vi "FXP_AFMss_MPC_singleAxis_N22.vi"() -> ()   [LabVIEW 2017]
uses:
  fpga_fp_interface_lib/fpga_interface_types/boolean_indicators.ctl
  fgm_pipiline/quadProgParams_pipe.ctl
  typeDefs/FXPControlParams_distEst.ctl
  <vilib>/rvi/eio/common/nirviEmuClasses.ctl
  <vilib>/Platform/TimedLoop/XDataNode/timing_clust.ctl
  <vilib>/Platform/TimedLoop/XDataNode/nitl_modes.ctl
  <vilib>/Platform/TimedLoop/XDataNode/wakeup.ctl
  <vilib>/rvi/Emulation/niFpgaSctlEmulationGetInTimedLoop.vi
  <vilib>/rvi/Emulation/niFpgaProcessEmulError.vi
  <vilib>/rvi/eio/common/nirviEmuTemplateMethod_errors.vi
  <vilib>/rvi/Emulation/niFpgaGetClockAttributes.vi
  <vilib>/rvi/Emulation/niFpgaEmulationReportErrorSimple.vi
  <vilib>/rvi/Emulation/niFpgaCriticalErrorInLSC.vi
  <vilib>/rvi/Memory/Memory_Emulation/nirvimemoryFastEmulation.vi
  <vilib>/rvi/Memory/Memory_Emulation/nirvimemoryEmulation.vi
  <vilib>/rvi/Emulation/niFpgaEmulationIsFPGAContextNoSignature.vi
  <vilib>/rvi/DataTransferAndStorage/Container/Common/niFpgaContainerGetUniqueNameForEmu.vi
  <vilib>/rvi/errors/nirviReportUnexpectedCaseInternalError (U32).vi
  <vilib>/rvi/interface/RandomDataEmulation/niFpgaRandomDataHandleErrors.vi
  <vilib>/eio/EIOGrowableMethodNode/genericMethod/EIOGrowableMethodNode.xnode
  <vilib>/rvi/eio/nirviEIOMethodImplementation/nirviEIOMethodImplementation.xnode
  <vilib>/rvi/eio/nirviErrorMerge/nirviErrorMerge.xnode
  <vilib>/eio/EIONode/EIONode.xnode
  <vilib>/Platform/TimedLoop/XDataNode/XDataNode.xnode
  <vilib>/rvi/DataTransferAndStorage/Container/XNode/niFpgaContainer.xnode
  <vilib>/rvi/interface/RandomDataEmulation/nirviRandomDataFpgaReadWriteTemplate.vi
  <vilib>/rvi/FXPMathLib/FxpSub/XNode/nifxpmath_Sub.xnode
  <vilib>/Platform/TimedLoop/XDataNode/XDNodeRunTimeDep.lvlib
  <vilib>/rvi/FXPMathLib/sim/FxpSim.dll
panel:
  in  "N_sat":i32
  in  "sat_d_s":fxp<+/-,16,5>[](array[numeric])=[0.0, 0.0, 0.0, 0.0, 0.0, 0.0, 0.0]
  in  "sat_w_s":fxp<+/-,16,5>[](array[numeric])=[0.0, 0.0, 0.0, 0.0, 0.0, 0.0, 0.0]
  out "fpga_debug":bool
  out "fpga_debug":bool
  in  "N_hyst":i32
  in  "w_s":fxp<+/-,16,5>[](array[numeric])=[0.0, 0.0, 0.0, 0.0, 0.0, 0.0, 0.0]
  in  "r_s":fxp<+/-,16,5>[](array[numeric])=[0.0, 0.0, 0.0, 0.0, 0.0, 0.0, 0.0]
  out "Ipow fast":fxp<+/-,16,5>
  in  "Num":sgl[](array[numeric])=[-0.00254, 0.000408, 0.00295, 0.0, 0.0, 0.0, 0.0, 0.0, 0.0]
  in  "Den":sgl[](array[numeric])=[0.982758, -1.98194, 1.0, 0.0, 0.0, 0.0, 0.0, 0.0, 0.0]
  in  "TF Order":i32=2
  out "y_ref":sgl
  in  "ControlParams_distEst":T1={"umax"=3.0, "Ns_obs/cntrl"=0, "ref_f_VEC"=[0.0, 0.0], "du_max"=0.0}
  in  "QP_params":T2={"maxIter"=0, "nuN"=24, "Ns_mpc"=0, "-beta"=-0.9987945556640625, "beta+1"=1.9987945556640625}
  out "Matrix FIFO \nTimeOut":bool
  out "u_k":fxp<+/-,32,5>
  out "boolean  indicators":T3
  out "x-x(0)":fxp<+/-,18,5>
  out "y-axis fast":fxp<+/-,16,5>
  out "x(0)":fxp<+/-,16,5>
  out "LoopTicks2":u32
  out "Error Out":errorcluster
  out "x-axis fast":fxp<+/-,16,5>
  out "AI Timed Out":bool
  out "Stopped":bool
  in  "Settle Ticks":i16=1000
  in  "iters":i32=1
  in  "ymax":fxp<+/-,32,16>=4.0
  in  "TsTicks":i16
  out "Loop Ticks (benchmark)":i16
  out "NS_O/C":u8=2
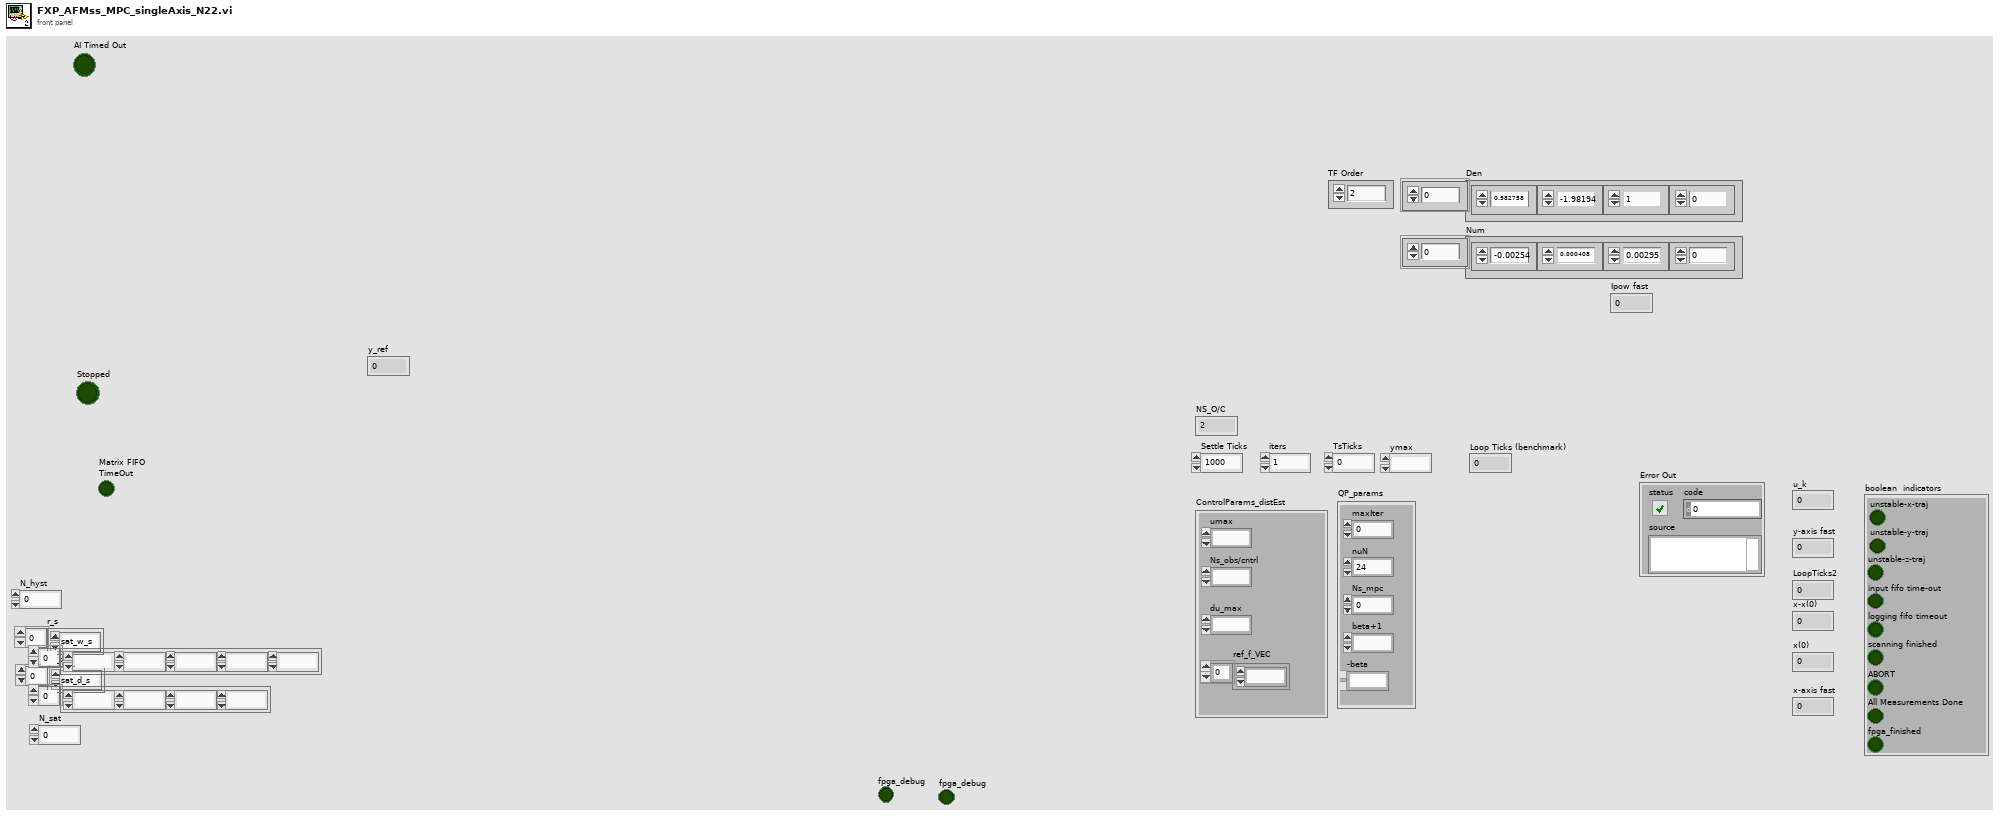
[diagram p1: front panel]
types:
  T1 = typedef "FXPControlParams_distEst.ctl" = cluster{"umax":fxp<+/-,18,5>, "Ns_obs/cntrl":u8, "ref_f_VEC":fxp<+/-,32,5>[], "du_max":fxp<+/-,18,5>}
  T2 = typedef "quadProgParams_pipe.ctl" = cluster{"maxIter":u16, "nuN":u16, "Ns_mpc":u16, "-beta":fxp<+/-,18,2>, "beta+1":fxp<+/-,18,2>}
  T3 = typedef "boolean_indicators.ctl" = cluster{"unstable-z-traj":bool, "input fifo time-out":bool, "logging fifo timeout":bool, "scanning finished":bool, "unstable-x-traj":bool, "unstable-y-traj":bool, "ABORT":bool, "All Measurements Done":bool, "fpga_finished":bool}
  T4 = typedef "nirviEmuClasses.ctl" = enum16{"IO Read", "IO Write", "Method", "Property Read", "Property Write"}
  T5 = typedef "XDNodeRunTimeDep.lvlib/timing_clust.ctl" = cluster{"Expected End [f-1]":u64, "Actual End [f-1]":u64, "Finished Late? [f-1]":bool, "Expected End [i-1]":u64, "Actual End [i-1]":u64, "Finished Late? [i-1]":bool, "Expected Start [i]":u64, "Actual Start [i]":u64, "Expected Start [f]":u64, "Actual Start [f]":u64, "Source Name":string, "Structure Name":string, "Period":i64, "Deadline":i64, "Offset":i64, "Start":i64, "Priority":i32, "Timeout":i32, "Mode":T6, "Wakeup Reason":T7, "Error":errorcluster, "Source Type":string, "Secondary Source Type":string, "Global End Time":u64, "Global Start Time":u64, "Frame Duration":u64, "Iteration Duration":u64, "Assigned CPU":i32, "I/O Scan Engine Mode":u32}
  T6 = typedef "XDNodeRunTimeDep.lvlib/nitl_modes.ctl" = enum32{"No Change", "Process missed periods, maintain original phase", "Discard missed periods, maintain original phase", "Process missed periods, ignore original phase", "Discard missed periods, ignore original phase"}
  T7 = typedef "XDNodeRunTimeDep.lvlib/wakeup.ctl" = enum32{"Normal", "Aborted", "Asynchronous wakeup", "Timing source error", "Timed loop error", "Timeout"}
  T8 = typedef "x_vec_type.ctl" = fxp<+/-,32,6>[]
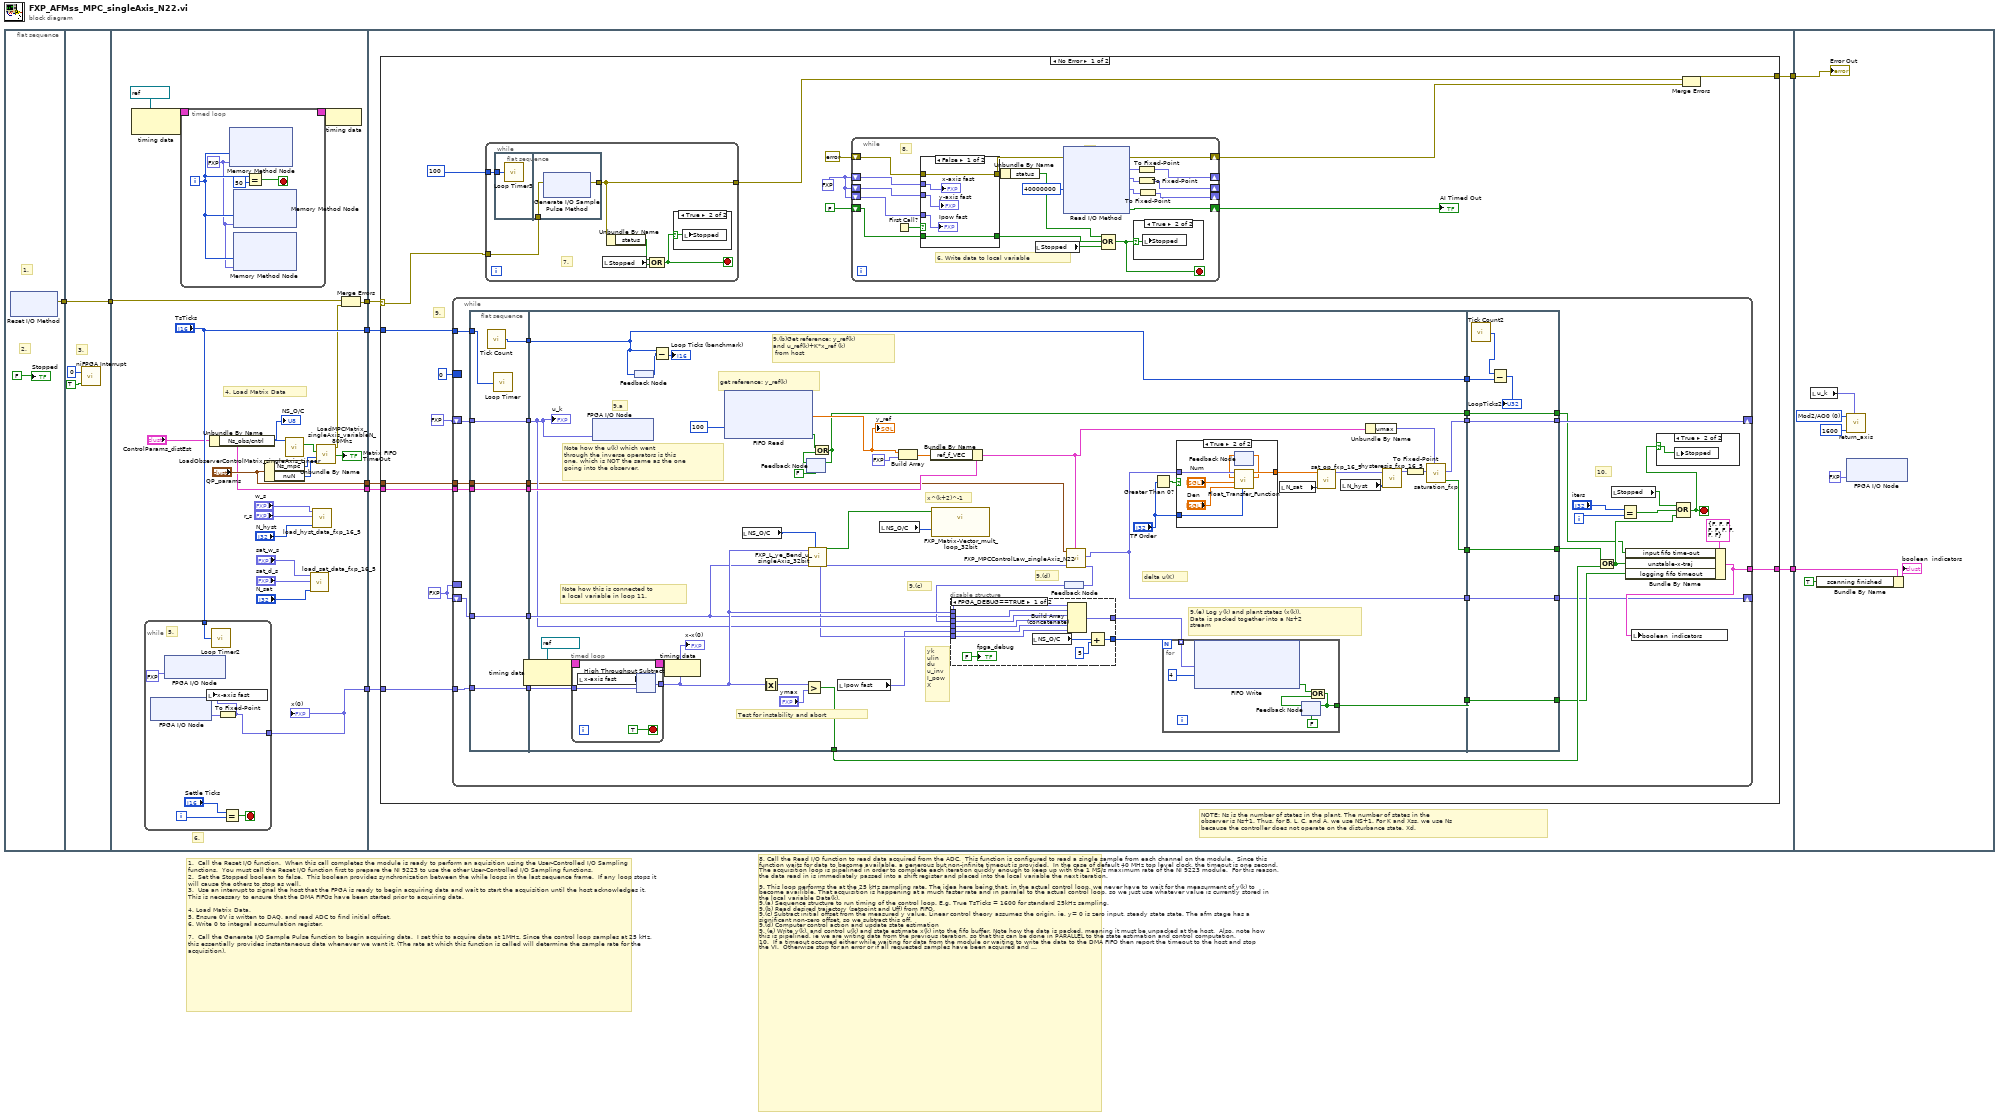
[diagram p0: block diagram]
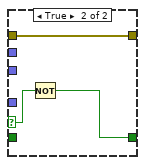
[diagram p2: hidden frame]
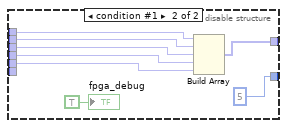
[diagram p6: hidden frame]
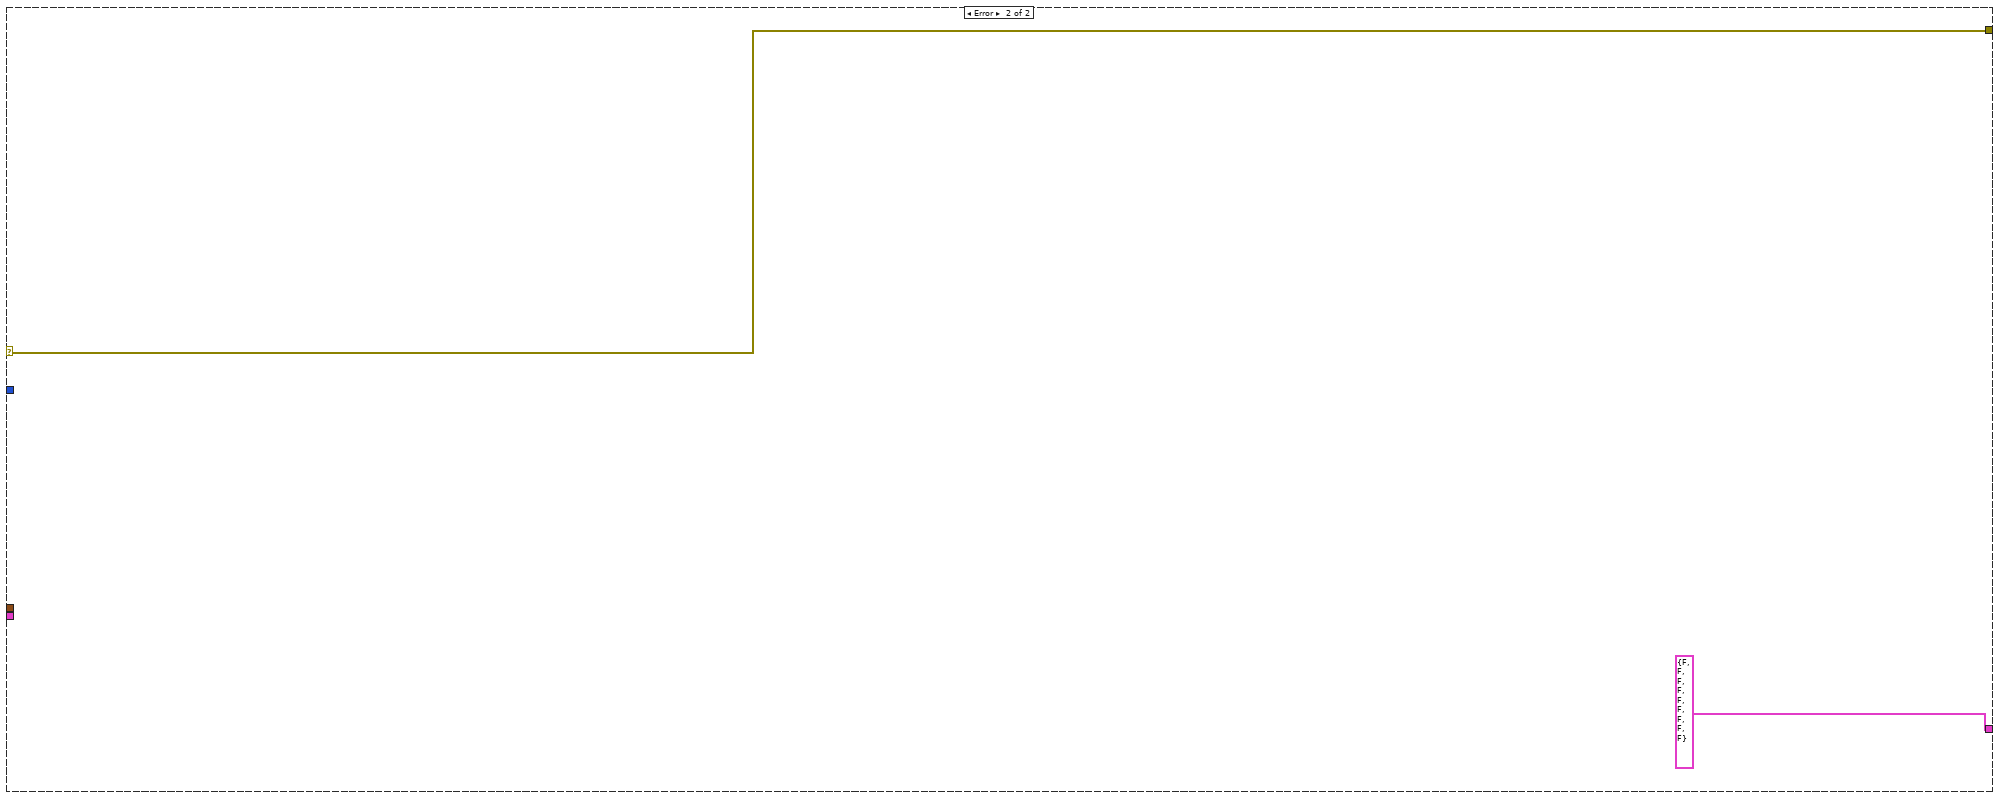
[diagram p8: hidden frame]
diagram:
  # "8. Call the Read I/O function to read data acquired from the ADC.  This function is configured to read a single sample from each channel on the module.  Since this function waits for data to become available, a generous but non-infinite timeout is provided.  In the case of default 40 MHz top level clock, the timeout is one second.  The acquisition loop is pipelined in order to complete each iteration quickly enough to keep up with the 1 MS/s maximum rate of the NI 9223 module.  For this reason, the data read in is immediately passed into a shift register and placed into the local variable the next iteration.\n\n9. This loop performs the at the 25 kHz sampling rate. The idea here being that, in the actual control loop, we never have to wait for the measurment of y(k) to become availible. That acquisition is happening at a much faster rate and in parralel to the actual control loop, so we just use whatever value is currently stored in the local variable Data(k).\n9.(a) Sequence structure to run timing of the control loop. E.g. True TsTicks = 1600 for standard 25kHz sampling.\n9.(b) Read desired trajectory (setpoint and Uff) from FIFO.\n9.(c) Subtract initial offset from the measured y value. Linear control theory assumes the origin, ie, y= 0 is zero input, steady state state. The afm stage has a significant non-zero offset, so we subtract this off.\n9.(d) Computer control action and update state estimation\n9. (e) Write y(k), and control u(k) and state estimate x(k) into the fifo buffer. Note how the data is packed, meaning it must be unpacked at the host.  Also, note how this is pipelined, ie we are writing data from the previous iteration, so that this can be done in PARALLEL to the state estimation and control computation.  \n10.  If a timeout occurred either while waiting for data from the module or waiting to write the data to the DMA FIFO then report the timeout to the host and stop the VI.  Otherwise stop for an error or if all requested samples have been acquired and placed into the DMA FIFO or if the controll law has detected instability.\n\n11. WRITE  TO DAQ. Note how the output of the control law is connected to loop 11 through a local variable."
  # "1.  Call the Reset I/O function.  When this call completes the module is ready to perform an aquisition using the User-Controlled I/O Sampling functions.  You must call the Reset I/O function first to prepare the NI 9223 to use the other User-Controlled I/O Sampling functions.\n2.  Set the Stopped boolean to false.  This boolean provides synchronization between the while loops in the last sequence frame.  If any loop stops it will cause the others to stop as well.\n3.  Use an interrupt to signal the host that the FPGA is ready to begin acquiring data and wait to start the acquisition until the host acknowledges it.  This is necessary to ensure that the DMA FIFOs have been started prior to acquiring data.\n\n4. Load Matrix Data.\n5. Ensure 0V is written to DAQ, and read ADC to find initial offset.\n6. Write 0 to integral accumulation register.\n\n7.  Call the Generate I/O Sample Pulse function to begin acquiring data.  I set this to acquire data at 1MHz. Since the control loop samples at 25 kHz, this essentially provides instantaneous data whenever we want it. (The rate at which this function is called will determine the sample rate for the acquisition)."
  n1 = flat-sequence {
    tunnel: [w10] -> w4
    tunnel: [w56] -> w5
    tunnel: w4 -> [w56]
    tunnel: ["TsTicks"] -> w9
    tunnel: [w79] -> w8
    tunnel: ["ControlParams_distEst"] -> w7
    tunnel: [w73] -> w6
    tunnel: w5 -> [w72]
    tunnel: ["QP_params"] -> w1
    tunnel: w9 -> [w103]
    tunnel: w8 -> [w102]
    tunnel: w7 -> [w101]
    tunnel: w6 -> [w100]
    tunnel: [w99] -> w3
    tunnel: [w98] -> w2
    tunnel: w1 -> [w97]
    tunnel: w3 -> [w495]
    tunnel: w2 -> [w493]
    frame #0 {
      # "2."
      # "1."
      n2 = xnode "Reset I/O Method"() -> ("error out"=w10:errorcluster)  [unwired: 2 in, 1 out]
      "Stopped" <- FALSE ("Stopped")
    }
    frame #1 {
      # "3."
      n3 = call <vilib>:"niFPGA Interrupt.vi"("Wait Until Cleared (F)"=TRUE, "IRQ Number (0)"=u8 0) -> ()  [unwired: 1 in]
    }
    frame #2 {
      # "6."
      # "4. Load Matrix Data"
      n4 = node-c288(refnum<k21> "80MHz" ("Source Name")) -> (w77:T5)
      n5 = while {
        tunnel: [w94] -> w79
        tunnel: "TsTicks" -> [w96]
        i -> [w90]
        stop <- w92 stop-if-true
        # "5."
        n6 = xnode "FPGA I/O Node"() -> ("Mod2/AI0"=w95:fxp<+/-,24,5>)  [unwired: 1 in, 1 out]
        n7 = xnode "FPGA I/O Node"("Mod1/AO0"=fxp<+,1,1> 0.0) -> ()  [unwired: 1 in, 1 out]
        n8 = call "Loop Timer2"("Count(Ticks)"=w96) -> ()  [unwired: 1 out]
        n9 = To Fixed-Point(number=w95) -> (fixed-point=w94:fxp<+/-,16,5>)  [unwired: 1 in]
        n10 = local write "x-axis fast"(w94) -> ()
        n11 = Equal?(x="Settle Ticks", y=w90) -> (x = y?=w92:bool)
      }
      "x(0)" <- w79
      n12 = timed-loop {
        timing: w77 -> [_]
        timing-out: [_] -> w76
        i -> [w81]
        stop <- w83 stop-if-true
        w80 = fxp<+/-,32,5> 0.0 ("Data")
        n13 = xnode ("Memory Method Node")("Address"=w81, "Data"=w80) -> ()  [unwired: 1 in, 1 out]
        n14 = xnode ("Memory Method Node")("Address"=w81, "Data"=w80) -> ()  [unwired: 1 in, 1 out]
        n15 = xnode ("Memory Method Node")("Address"=w81, "Data"=w80) -> ()  [unwired: 1 in, 1 out]
        n16 = Equal?(x=w81, y=50) -> (x = y?=w83:bool)
      }
      n17 = Unbundle By Name("ControlParams_distEst") -> ("Ns_obs/cntrl"=w74:u8)
      "NS_O/C" <- w74
      n18 = Unbundle By Name("QP_params") -> ("Ns_mpc"=w60:u16, "nuN"=w61:u16)
      n19 = call "LoadObserverControlMatrix_singleAxis_Linear.vi"("NS_obs/cntrl"=w74) -> ("SS FIFO TimeOut?"=w59:bool)  [unwired: 10 in]
      n20 = call "load_sat_data_fxp_16_5.vi"("N_sat"="N_sat", "sat_d_s"="sat_d_s", "sat_w_s"="sat_w_s") -> ()  [unwired: 9 in]
      n21 = call "load_hyst_data_fxp_16_5.vi"("N_hyst"="N_hyst", "r_s"="r_s", "w_s"="w_s") -> ()  [unwired: 9 in]
      n22 = call "LoadMPCMatrix_singleAxis_variableN_80Mhz.vi"("nuN_mpc"=w61, "Ns+1"=w60, "FIFO Timeout\nIn"=w59) -> ("FIFO Matrix Timeout"=→"Matrix FIFO \nTimeOut":bool, "error out"=w63:errorcluster)  [unwired: 7 in]
      n23 = node-c288(w76) -> ()
      n24 = Merge Errors(w72, w63) -> (w73:errorcluster)
    }
    frame #3 {
      # "NOTE: Ns is the number of states in the plant. The number of states in the \nobserver is Ns+1. Thus, for B, L, C, and A, we use NS+1. For K and Xss, we use Ns\nbecause the controller does not operate on the disturbance state, Xd."
      n25 = case shown="No Error" w100 {
        selector: w100 -> [w110 w487]
        tunnel: w103 -> [w111 _]
        tunnel: w102 -> [w112 _]
        tunnel: w101 -> [w119 _]
        tunnel: [w116 w487] -> w99
        tunnel: [w109 T3 {"unstable-z-traj"=FALSE, "input fifo time-out"=FALSE, "logging fifo timeout"=FALSE, "scanning finished"=FALSE, "unstable-x-traj"=FALSE, "unstable-y-traj"=FALSE, "ABORT"=FALSE, "All Measurements Done"=FALSE, "fpga_finished"=FALSE} ("boolean  indicators 2")] -> w98
        tunnel: w97 -> [w107 _]
        frame No Error {
          w105 = fxp<+/-,18,5> 0.0
          w104 = fxp<+/-,16,5> 0.0 ("Mod1/AI0")
          # "9."
          n26 = while {
            border: i16 0 -> [_]
            tunnel: w119 -> [w377]
            shift-right: [w366] -> _
            shift-left: fxp<+/-,18,5> 0.0 -> [w349]
            tunnel: w112 -> [w375]
            tunnel: w111 -> [w367]
            border: w105 -> [_]
            tunnel: [w361] -> w109
            tunnel: w107 -> [w355]
            shift-right: [w351] -> _
            shift-left: w105 -> [w348]
            i -> [w378]
            stop <- w358 stop-if-true
            # "10."
            n27 = flat-sequence {
              tunnel: w375 -> [w385]
              tunnel: w348 -> [w386]
              tunnel: w377 -> [w387]
              tunnel: [w387] -> w371
              tunnel: [w386] -> w370
              tunnel: [w385] -> w369
              tunnel: [w384] -> w368
              tunnel: w367 -> [w383]
              tunnel: [w382] -> w356
              tunnel: w355 -> [w382]
              tunnel: [w381] -> w350
              tunnel: w349 -> [w381]
              tunnel: [w433] -> w362
              tunnel: [w400] -> w374
              tunnel: [w434] -> w373
              tunnel: [w432] -> w372
              tunnel: w368 -> [w432]
              tunnel: w369 -> [w425]
              tunnel: w370 -> [w407]
              tunnel: w371 -> [w417]
              tunnel: [w399] -> w365
              tunnel: w356 -> [w391]
              tunnel: [w408] -> w354
              tunnel: [w388] -> w352
              tunnel: w350 -> [w406]
              tunnel: [w485] -> w357
              tunnel: w374 -> [w481]
              tunnel: w373 -> [w485]
              tunnel: w372 -> [w483]
              tunnel: [w481] -> w366
              tunnel: [w480] -> w363
              tunnel: w365 -> [w480]
              tunnel: w354 -> [w479]
              tunnel: [w479] -> w353
              tunnel: w352 -> [w478]
              tunnel: [w478] -> w351
              frame #0 {
                n28 = call "Tick Count"() -> ("Tick Count(Ticks)"=w384:u32)
                n29 = call "Loop Timer"("Count(Ticks)"=w383) -> ()  [unwired: 1 out]
              }
              frame #1 {
                # "yk\nulin\ndu\nu_inv\nI_pow\nX"
                # "Note how the u(k) which went \nthrough the inverse operators is this\none, which is NOT the same as the one\ngoing into the observer."
                # "get reference: y_ref(k)"
                # "delta u(K)"
                # "Note how this is connected to\na local variable in loop 11."
                # "9.a"
                # "x^(k+2)^-1"
                # "9.(c)"
                # "9.(b)Get reference: y_ref(k)\nand u_ref(k)+K*x_ref (k)\n from host"
                # "9.(d)"
                # "9.(e) Log y(k) and plant states (x(k)). \nData is packed together into a Ns+2 \nstream"
                # "Test for instability and abort"
                n30 = node-c288(refnum<k21> "80MHz" ("Source Name")) -> (w429:T5)
                n31 = timed-loop {
                  timing: w429 -> [_]
                  timing-out: [_] -> w428
                  tunnel: w425 -> [w464]
                  tunnel: [w463] -> w422
                  stop <- TRUE stop-if-true
                  n32 = local read "x-axis fast"() -> (w465:fxp<+/-,16,5>)
                  n33 = xnode "High Throughput Subtract"("x"=w465, "y"=w464) -> ("x-y"=w463:fxp<+/-,18,5>)
                }
                "x-x(0)" <- w422
                n34 = xnode "FPGA I/O Node"("Mod1/AO0"=w406) -> ()  [unwired: 1 in, 1 out]
                n35 = feedback #1() -> (w426:u32)
                n36 = feedback-in #1(w432) -> ()
                n37 = Subtract(x=w432, y=w426) -> (x-y=→"Loop Ticks (benchmark)":u32)
                n38 = node-c288(w428) -> ()
                n39 = xnode ("FIFO Read")("Timeout"=i16 100) -> ("Element"=w414:sgl, "Timed Out?"=w409:bool)  [unwired: 1 in, 1 out]
                "y_ref" <- w414
                n40 = local read "NS_O/C"() -> (w404:u8)
                n41 = Absolute Value(x=w422) -> (abs(x)=w431:fxp<+,18,5>)
                n42 = Greater?(x=w431, y="ymax") -> (0:w433:bool)
                n43 = feedback #2(FALSE) -> (w410:bool)
                n44 = call "FXP_L_ye_Bend_u_singleAxis_32bit.vi"("NS"=w404, "U(k): ux"=w407, "Y(k): x"=w422) -> ("yd_est"=w390:fxp<+/-,32,5>, "outputValid"=w423:bool, "x0"=w405:T8)  [unwired: 6 in]
                n45 = Or(x=w409, y=w410) -> (x .or. y?=w408:bool)
                n46 = feedback-in #2(w408) -> ()
                n47 = local read "Ipow fast"() -> (w402:fxp<+/-,16,5>)
                n48 = local read "NS_O/C"() -> (w403:u8)
                n49 = Build Array(w414, fxp<+,1,1> 0.0) -> (w416:sgl[])
                n50 = Bundle By Name(cluster=w417, "ref_f_VEC"=w416) -> (w392:T1)
                n51 = call "FXP_Matrix-Vector_mult_loop_32bit.vi"("Ns_2"=w403, "inputValid"=w423) -> ()  [unwired: 9 in, 1 out]
                n52 = feedback #3() -> (w421:fxp<+/-,64,15>)
                n53 = disable-structure shown="FPGA_DEBUG==TRUE" {
                  disable-tunnel: w422 -> [w445 w451]
                  disable-tunnel: w421 -> [w444 w449]
                  disable-tunnel: [w443 w452] -> w420
                  disable-tunnel: [w441 u8 5 ("y")] -> w419
                  disable-tunnel: w407 -> [w440 w450]
                  disable-tunnel: w406 -> [w439 w448]
                  disable-tunnel: w405 -> [w438 _]
                  disable-tunnel: w402 -> [w436 w447]
                  frame condition #0 (active) {
                    n54 = local read "NS_O/C"() -> (w437:u8)
                    n55 = Build Array (concatenate)(w445, w440, w444, w439, w436, w438) -> (w443:fxp<+/-,64,15>[])
                    n56 = Add(x=w437, y=u8 5) -> (x+y=w441:u8)
                    "fpga_debug" <- FALSE
                  }
                  frame condition #1 {
                    n57 = Build Array(w451, w450, w449, w448, w447) -> (w452:fxp<+/-,64,15>[])
                    "fpga_debug" <- TRUE
                  }
                }
                n58 = call "FXP_MPCControlLaw_singleAxis_N22.vi"("ControlParams_distEst"=w392, "yd_est_x"=w390, "QP_params"=w391) -> ("del u_x"=w389:fxp<+/-,64,15>, "u_k (un saturated)"=w388:fxp<+/-,32,5>)  [unwired: 7 in]
                n59 = feedback-in #3(w389) -> ()
                n60 = Greater Than 0?(x="TF Order") -> (x > 0?=w413:bool)
                n61 = for {
                  N: w419 -> [_]
                  tunnel: w420 -> [w476] mode=indexing
                  tunnel: [w472] -> w434
                  n62 = xnode ("FIFO Write")("Element"=w476, "Timeout"=i16 4) -> ("Timed Out?"=w475:bool)  [unwired: 1 in, 1 out]
                  n63 = feedback #4(FALSE) -> (w474:bool)
                  n64 = Or(x=w475, y=w474) -> (x .or. y?=w472:bool)
                  n65 = feedback-in #4(w472) -> ()
                }
                n66 = case shown="True" w413 {
                  tunnel: w388 -> [w454 w461]
                  tunnel: "TF Order" -> [_ w460]
                  tunnel: [w454 w459] -> w395
                  frame False {
                  }
                  frame True {
                    n67 = feedback #5() -> (w457:sgl[])  [unwired: 1 in]
                    n68 = call "Float_Transfer_Function.vi"("TF Order"=w460, "Den"="Den", "Num"="Num", "State In"=w457, "Input"=w461) -> ("State Out"=w458:sgl[], "Output"=w459:sgl)  [unwired: 4 in]
                    n69 = feedback-in #5(w458) -> ()
                  }
                }
                n70 = local read "N_sat"() -> (w393:i32)
                n71 = call "sat_op_fxp_16_5.vi"("N_sat"=w393, "uk_in"=w395) -> ("Hinv(uk)"=w394:fxp<+/-,32,10>)  [unwired: 9 in]
                n72 = local read "N_hyst"() -> (w401:i32)
                n73 = Unbundle By Name(w392) -> ("umax"=w397:fxp<+/-,18,5>)
                n74 = call "hysteresis_fxp_16_5.vi"("N_hyst"=w401, "uk_in"=w394) -> ("Hinv(uk)"=w396:fxp<+/-,32,10>)  [unwired: 9 in]
                n75 = To Fixed-Point(number=w396) -> (fixed-point=w398:fxp<+/-,32,5>)  [unwired: 1 in]
                n76 = call "saturation_fxp.vi"("uMax"=w397, "signal_in"=w398) -> ("has_saturated"=w399:bool, "signal_out (saturated)"=w400:fxp<+/-,32,6>)  [unwired: 8 in]
                "u_k" <- w406
              }
              frame #2 {
                n77 = call "Tick Count2"() -> ("Tick Count(Ticks)"=w484:u32)
                n78 = Subtract(x=w484, y=w483) -> (x-y=→"LoopTicks2":u32)
              }
            }
            n79 = Or(x=w363, y=w362) -> (x .or. y?=w359:bool)
            n80 = local read "Stopped"() -> (w360:bool)
            n81 = Equal?(x="iters", y=w378) -> (x = y?=w376:bool)
            n82 = Bundle By Name(cluster=T3 {"unstable-z-traj"=FALSE, "input fifo time-out"=FALSE, "logging fifo timeout"=FALSE, "scanning finished"=FALSE, "unstable-x-traj"=FALSE, "unstable-y-traj"=FALSE, "ABORT"=FALSE, "All Measurements Done"=FALSE, "fpga_finished"=FALSE} ("boolean  indicators"), "input fifo time-out"=w353, "unstable-x-traj"=w359, "logging fifo timeout"=w357) -> (w361:T3)
            n83 = local write "boolean  indicators"(w361) -> ()
            n84 = Compound Arithmetic op=OR(w360, w376, w359) -> (w358:bool)
            n85 = case shown="True" w358 {
              selector: w358 -> [_ w380]
              frame False {
              }
              frame True {
                n86 = local write "Stopped"(w380) -> ()
              }
            }
          }
          n87 = while {
            tunnel: u32 100 ("Max TsTicks") -> [w299]
            tunnel: [w296] -> w114
            tunnel: w110 -> [w294]
            stop <- w295 stop-if-true
            # "7."
            n88 = flat-sequence {
              tunnel: w299 -> [w301]
              tunnel: [w303] -> w296
              tunnel: w294 -> [w302]
              frame #0 {
                n89 = call "Loop Timer3"("Count(Ticks)"=w301) -> ()  [unwired: 1 out]
              }
              frame #1 {
                n90 = xnode "Generate I/O Sample Pulse Method"("error in"=w302) -> ("error out"=w303:errorcluster)  [unwired: 1 in, 1 out]
              }
            }
            n91 = local read "Stopped"() -> (w298:bool)
            n92 = Unbundle By Name(w296) -> ("status"=w297:bool)
            n93 = Compound Arithmetic op=OR(w297, w298) -> (w295:bool)
            n94 = case shown="True" w295 {
              selector: w295 -> [_ w300]
              frame False {
              }
              frame True {
                n95 = local write "Stopped"(w300) -> ()
              }
            }
          }
          n96 = while {
            shift-right: [w139] -> w113
            shift-left: errorcluster {"status"=FALSE, "code"=0, "source"=""} ("error out") -> [w133]
            shift-right: [w138] -> w115
            shift-left: FALSE ("Timed Out") -> [w130]
            shift-right: [w128] -> _
            shift-left: w104 -> [w134]
            shift-right: [w127] -> _
            shift-left: w104 -> [w126]
            shift-right: [w122] -> _
            shift-left: w104 -> [w121]
            stop <- w137 stop-if-true
            # "8."
            # "6. Write data to local variable"
            # "5."
            n97 = First Call?() -> (First Call?: T/F=w131:bool)
            n98 = case shown="False" w131 {
              selector: w131 -> [_ w147]
              tunnel: [w143 w146] -> w135
              tunnel: w134 -> [w144 _]
              tunnel: w133 -> [w145 w148]
              tunnel: [w145 w148] -> w125
              tunnel: w130 -> [w143 _]
              tunnel: w126 -> [w142 _]
              tunnel: w121 -> [w141 _]
              frame False {
                "x-axis fast" <- w144
                "y-axis fast" <- w142
                "Ipow fast" <- w141
              }
              frame True {
                n99 = Not(x=w147) -> (.not. x?=w146:bool)
              }
            }
            n100 = Unbundle By Name(w125) -> ("status"=w132:bool)
            n101 = local read "Stopped"() -> (w136:bool)
            n102 = xnode "Read I/O Method"("error in"=w125, "Timeout"=40000000) -> ("error out"=w139:errorcluster, "Mod2/AI0"=w129:fxp<+/-,24,5>, "Mod2/AI1"=w124:fxp<+/-,24,5>, "Mod2/AI2"=w123:fxp<+/-,24,5>, "Timed Out"=w138:bool)  [unwired: 3 in, 3 out]
            n103 = Compound Arithmetic op=OR(w132, w135, w136) -> (w137:bool)
            n104 = case shown="True" w137 {
              selector: w137 -> [_ w149]
              frame False {
              }
              frame True {
                n105 = local write "Stopped"(w149) -> ()
              }
            }
            n106 = To Fixed-Point(number=w129) -> (fixed-point=w128:fxp<+/-,16,5>)  [unwired: 1 in]
            n107 = To Fixed-Point(number=w124) -> (fixed-point=w127:fxp<+/-,16,5>)  [unwired: 1 in]
            n108 = To Fixed-Point(number=w123) -> (fixed-point=w122:fxp<+/-,16,5>)  [unwired: 1 in]
          }
          "AI Timed Out" <- w115
          n109 = Merge Errors(w114, w113) -> (w116:errorcluster)
        }
        frame Error {
        }
      }
    }
    frame #4 {
      w490 = i16 0 items=["Mod2/AO0", "Mod2/AO1", "Mod2/AO2", "Mod2/AO3", ""] ("DAC-select")
      n110 = local read "u_k"() -> (w488:fxp<+/-,32,5>)
      n111 = Bundle By Name(cluster=w493, "scanning finished"=TRUE) -> (→"boolean  indicators":T3)
      n112 = xnode "FPGA I/O Node"("Mod1/AO1"=fxp<+/-,20,5> 0.0 ("Mod1/AO0")) -> ()  [unwired: 1 in, 1 out]
      n113 = call "return_axis.vi"("u(0)"=w488, "TsTicks"=u32 1600, "DAC-select"=w490) -> ()  [unwired: 9 in]
      "Error Out" <- w495
    }
  }
